vi "HexSequenceStringDER.vi"(1 "Hex(sequence)":string) -> (0 "DER":string)   [LabVIEW 2023]
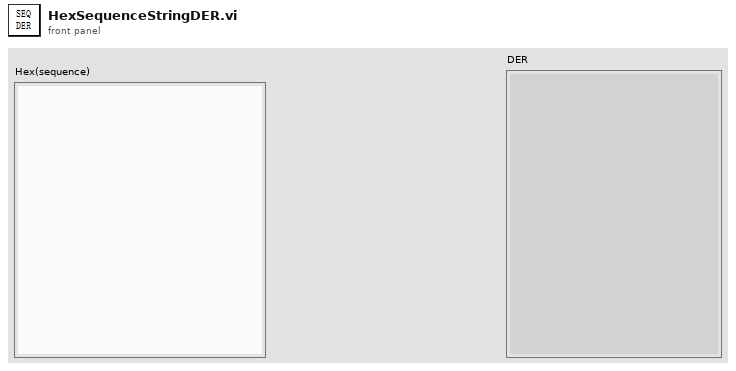
[diagram p1: front panel]
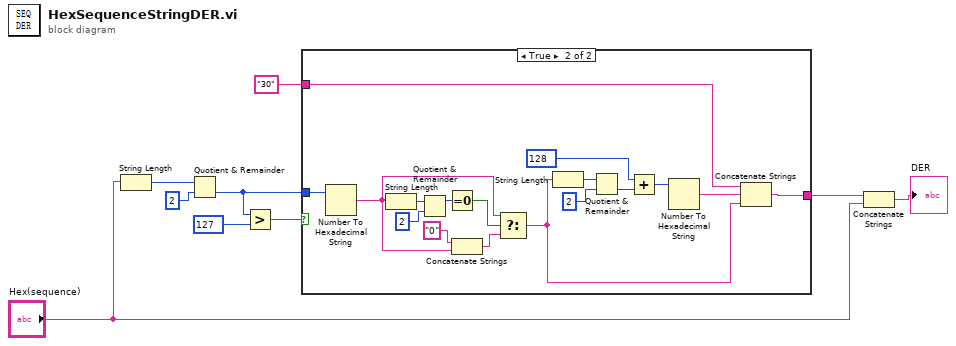
[diagram p0: block diagram]
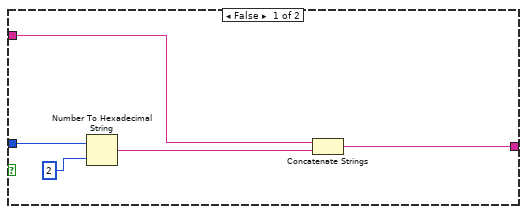
[diagram p2: hidden frame]
diagram:
  n1 = String Length(string="Hex(sequence)") -> (length=w9:i32)
  n2 = Quotient & Remainder(x=w9, y=2) -> (floor(x/y)=w5:i32)  [unwired: 1 out]
  n3 = Greater?(x=w5, y=127) -> (0:w6:bool)
  n4 = case shown="True" w6 {
    tunnel: w5 -> [w14 w30]
    tunnel: "30" -> [w13 w18]
    tunnel: [w11 w16] -> w3
    frame False {
      n5 = Number To Hexadecimal String(1:2, 2:w14) -> (0:w12:string)
      n6 = Concatenate Strings(w13, w12) -> (w11:string)
    }
    frame True {
      n7 = Number To Hexadecimal String(2:w30) -> (0:w23:string)  [unwired: 1 in]
      n8 = String Length(string=w23) -> (length=w26:i32)
      n9 = Quotient & Remainder(x=w26, y=2) -> (x-y*floor(x/y)=w27:i32)  [unwired: 1 out]
      n10 = Equal To 0?(x=w27) -> (x = 0?=w28:bool)
      n11 = Concatenate Strings("0", w23) -> (w29:string)
      n12 = Select(t=w23, s=w28, f=w29) -> (s? t:f=w15:string)
      n13 = String Length(string=w15) -> (length=w22:i32)
      n14 = Quotient & Remainder(x=w22, y=2) -> (floor(x/y)=w20:i32)  [unwired: 1 out]
      n15 = Add(x=128, y=w20) -> (x+y=w19:i32)
      n16 = Number To Hexadecimal String(2:w19) -> (0:w17:string)  [unwired: 1 in]
      n17 = Concatenate Strings(w18, w17, w15) -> (w16:string)
    }
  }
  n18 = Concatenate Strings(w3, "Hex(sequence)") -> (→"DER":string)
